vi "rm.server.visualize.close.vi"(8 "error in (no error)":errorcluster, 10 "Queue in":refnum<queue>, 11 "reference":refnum<vi>) -> (0 "error out":errorcluster)   [LabVIEW 2016, in "RM.Server.lvlib"]
uses:
  RM.Server.lvlib
  viz_command.ctl
  viz_state.ctl
  Shared/Global Tags.vi
  Shared/RM.Shared.lvlib
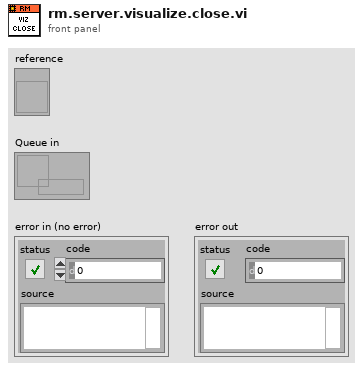
[diagram p1: front panel]
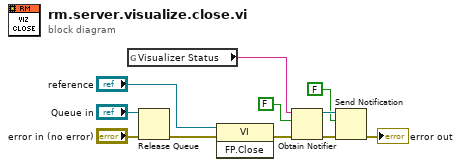
[diagram p0: block diagram]
diagram:
  n1 = global read "Global Tags.vi" "Visualizer Status"() -> (w7:string)
  n2 = Release Queue(queue="Queue in", error in (no error)="error in (no error)") -> (error out=w11:errorcluster)  [unwired: 1 in, 2 out]
  n3 = invoke class="VI" method="FP.Close"(reference="reference", error in=w11) -> (error out=w2:errorcluster)  [unwired: 1 in, 2 out]
  n4 = Obtain Notifier(name (unnamed)=w7, notification data type=FALSE, error in (no error)=w2) -> (notifier out=w5:refnum<notifier>, error out=w3:errorcluster)  [unwired: 1 in, 1 out]
  n5 = Send Notification(notification=FALSE, notifier=w5, error in (no error)=w3) -> (error out=→"error out":errorcluster)  [unwired: 1 out]
